vi "wavelength_GUI.vi"(4 "error in (no error)":errorcluster, 7 "connection ID":refnum<k5>) -> (0 "error out":errorcluster)   [LabVIEW 2015]
doc: "Use this template to build a PDA VI for Pocket PC 2002 devices or emulators."
panel:
  in  "Move Type":u16(ring) items=["BOTH", "GRATING ONLY", "CAMERA ONLY"]
  in  "Grating Angle":dbl min=0.0 max=5000.0
  in  "Cancel":bool
  in  "OK":bool
  in  "Camera Angle":dbl min=0.0 max=5000.0
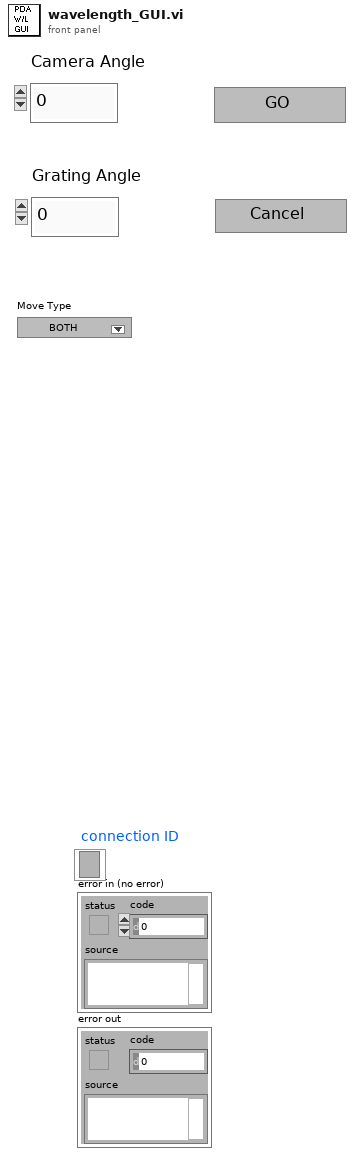
[diagram p1: front panel]
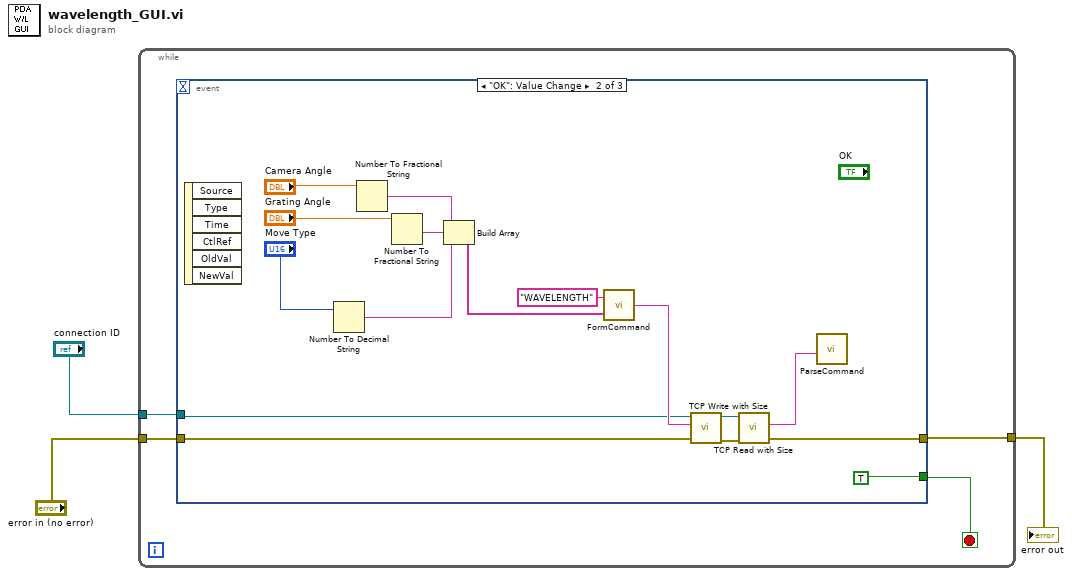
[diagram p0: block diagram]
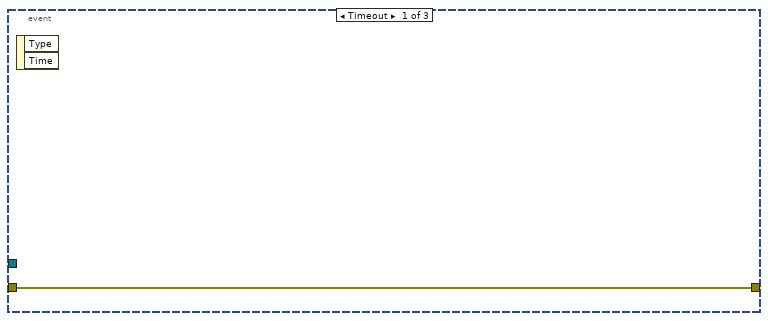
[diagram p2: hidden frame]
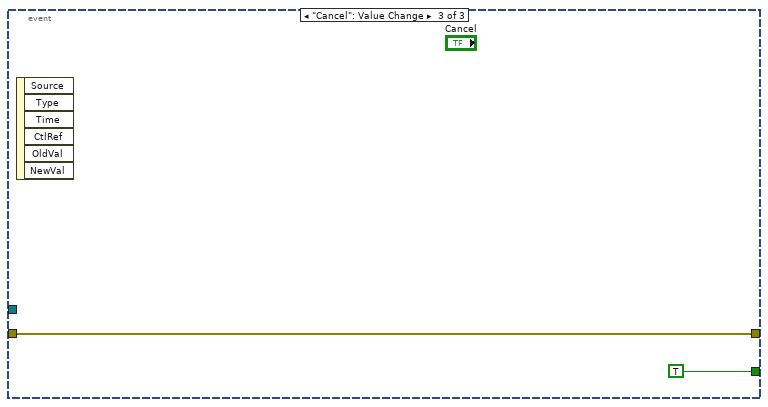
[diagram p3: hidden frame]
diagram:
  n1 = while {
    tunnel: "connection ID" -> [w7]
    tunnel: "error in (no error)" -> [w6]
    tunnel: [w5] -> w1
    stop <- w4 stop-if-true
    n2 = event shown="[1] \"OK\": Value Change" {
      selector: _ -> [_ _ _]
      dyn-events: _ -> [_ _ _]
      timeout: _ -> [_ _ _]
      tunnel: w7 -> [_ w10 _]
      tunnel: w6 -> [w8 w11 w26]
      tunnel: [w8 w9 w26] -> w5
      tunnel: [_ TRUE TRUE] -> w4
      event Timeout {
        n3 = event-data() -> ()  [unwired: 1 in, 2 out]
      }
      event "OK": Value Change {
        n4 = event-data() -> ()  [unwired: 1 in, 6 out]
        n5 = Number To Decimal String(number="Move Type") -> (decimal integer string=w19:string)  [unwired: 1 in]
        n6 = Number To Fractional String(number="Camera Angle") -> (F-format string=w20:string)  [unwired: 3 in]
        n7 = Number To Fractional String(number="Grating Angle") -> (F-format string=w18:string)  [unwired: 3 in]
        n8 = Build Array(w20, w18, w19) -> (w12:string[])
        n9 = call "FormCommand.vi"("Parameters"=w12, "Command"="WAVELENGTH") -> ("Command string"=w16:string)
        n10 = call "TCP Write with Size.vi"("error in (no error)"=w11, "data in"=w16, "connection ID"=w10) -> ("error out"=w13:errorcluster, "connection ID out"=w15:refnum<k5>)  [unwired: 6 in, 1 out]
        n11 = call "TCP Read with Size.vi"("error in (no error)"=w13, "connection ID"=w15) -> ("error out"=w9:errorcluster, "data out"=w14:string)  [unwired: 7 in, 1 out]
        n12 = call "ParseCommand.vi"("Command string"=w14) -> ()  [unwired: 2 out]
      }
      event "Cancel": Value Change {
        n13 = event-data() -> ()  [unwired: 1 in, 6 out]
      }
    }
  }
  "error out" <- w1
